vi "ZE_Recorder_CreateTask.vi"(8 "error in":errorcluster, 9 "multi device":bool, 11 "Channel Array In":T1 {"Terminal" items=["Default"=-1, "RSE"=10083, "NRSE"=10078, "Differential"=10106, "Pseudodifferential"=12529]}) -> (0 "error out":errorcluster, 1 "max Range":dbl, 2 "Task Array":refnum<k21>[](array[refnum]), 3 "Channel Array Out":T1 {"Terminal" items=["Default"=-1, "RSE"=10083, "NRSE"=10078, "Differential"=10106, "Pseudodifferential"=12529]})   [LabVIEW 2025, in "ZE_Recorder.lvlib"]
doc: "ZE_Recorder_CreateTask.vi\n----------------------------------------------\nThe VI creates the individual AI or temp tasks and asigns range and teriminal configuration.\nThe channels are assigned to as many tasks as needed.\n\nInputs:\n---------------------\n- error in : Cluster; \n- Channel Array : 1DArrayOfCluster; \n\nOutputs:\n---------------------\n- error out : Cluster; \n- task out : Refnum; \n- Channel Array : 1DArrayOfCluster; \n\n----------------------------------------------\n24.08.2016\nZühlke Engineering AG\nCH-8952 Schlieren\nwww.zuehlke.com"
uses:
  ZE_Recorder.lvlib
  ZE_Recorder_ChannelCluster.ctl
  ChannelCluster.ctl
  ZE_Recorder_Units.ctl
  Temperature.ctl
panel:
  # "Connector Pane"
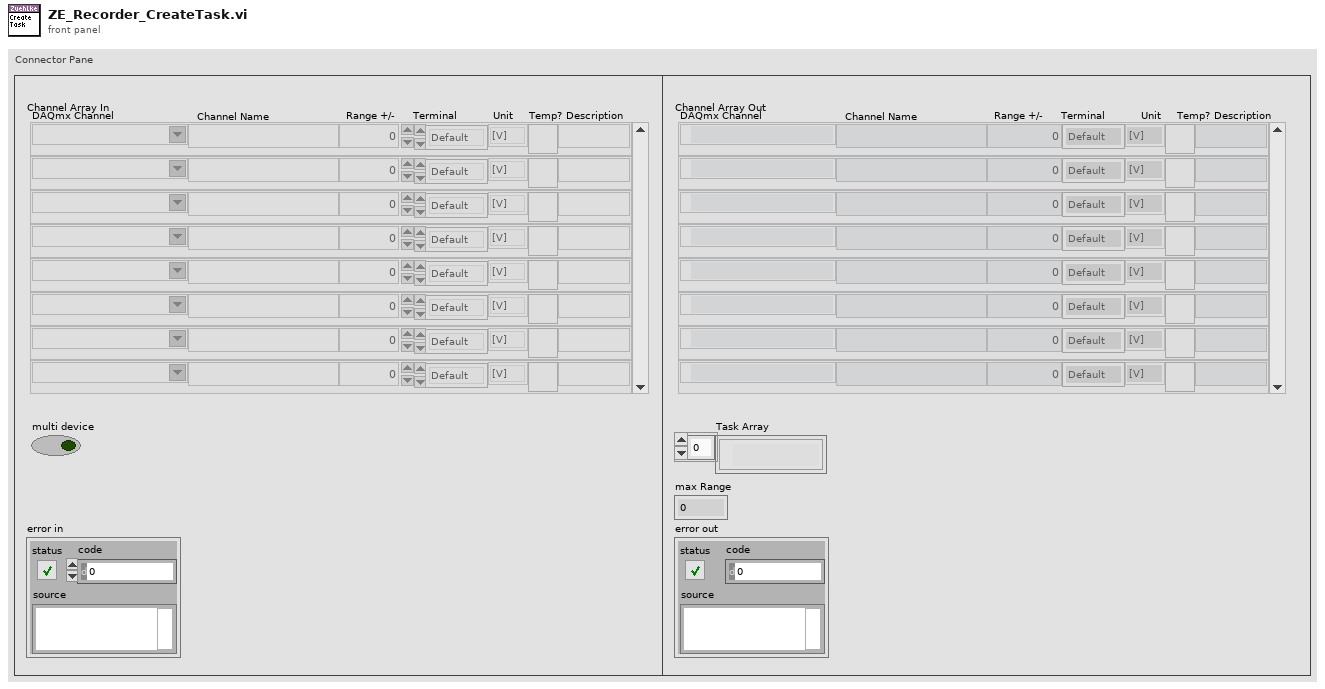
[diagram p1: front panel]
types:
  T1 = typedef "ZE_Recorder.lvlib/ZE_Recorder_ChannelCluster.ctl" = T2[]
  T2 = typedef "ZE_Recorder.lvlib/ChannelCluster.ctl" = cluster{"physical channel":tag, "channel name":string, "Range":dbl, "Terminal":i32, "Unit":T3, "isTemp":T4, "Description":string}
  T3 = typedef "ZE_Recorder.lvlib/ZE_Recorder_Units.ctl" = enum16{"[V]", "[A]", "[F]", "[H]", "[°C]", "[ml/s]", "[m/s]", "[bar]", "[%]", "[N]", "[?]"}
  T4 = typedef "ZE_Recorder.lvlib/Temperature.ctl" = bool
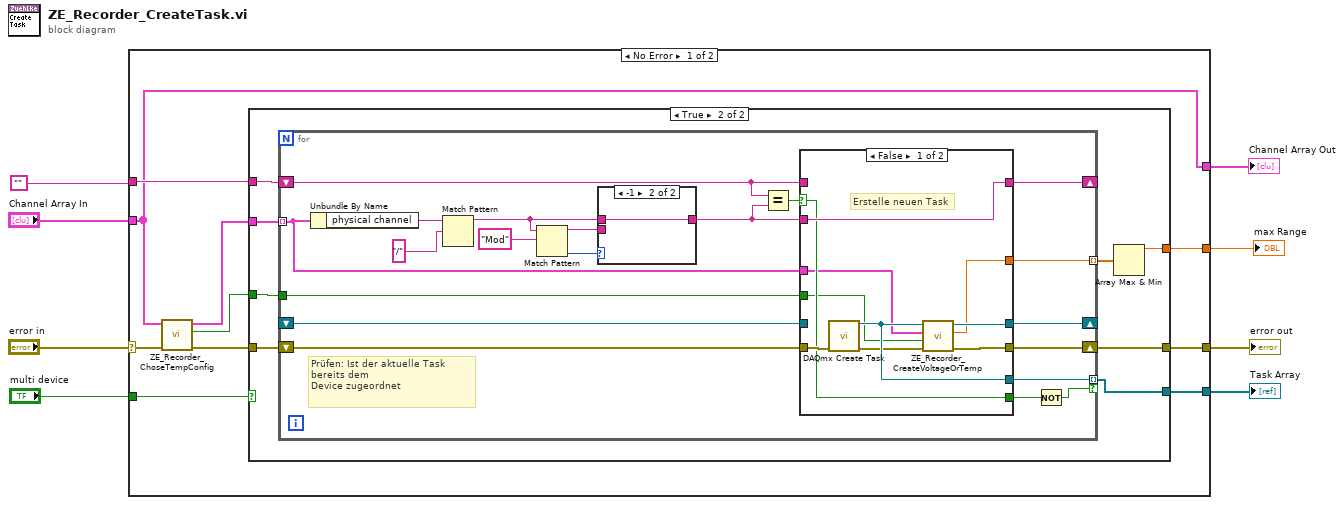
[diagram p0: block diagram]
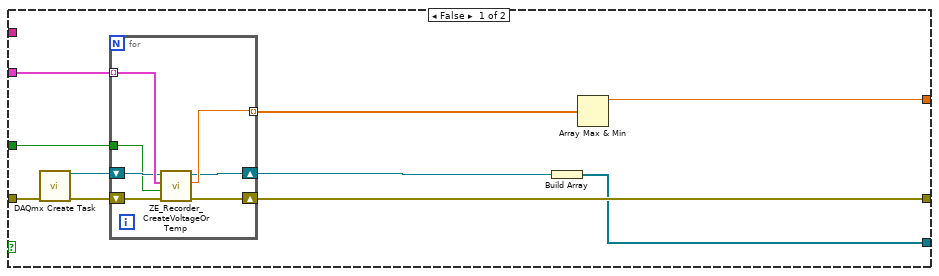
[diagram p2: hidden frame]
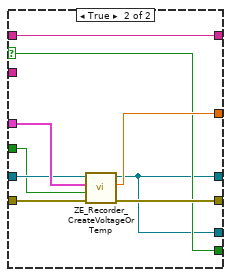
[diagram p4: hidden frame]
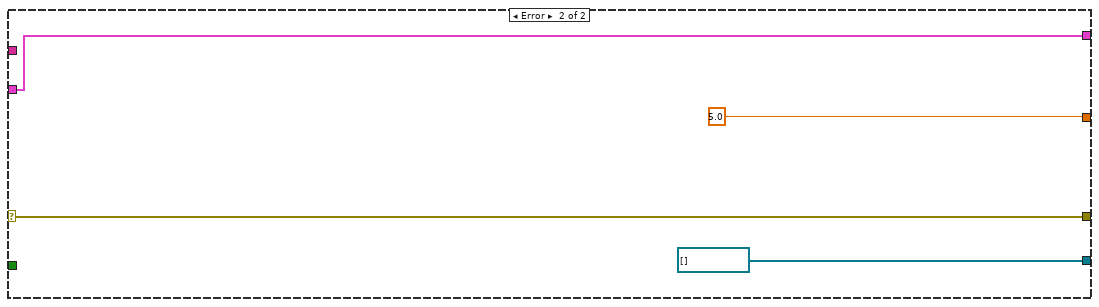
[diagram p5: hidden frame]
diagram:
  n1 = case shown="No Error" "error in" {
    selector: "error in" -> [w11 w87]
    tunnel: "Channel Array In" -> [w13 w88]
    tunnel: [w18 refnum<k21>[] []] -> w5
    tunnel: [w17 w87] -> w6
    tunnel: [w13 w88] -> w4
    tunnel: [w16 5.0] -> w3
    tunnel: "multi device" -> [w15 _]
    tunnel: "" -> [w14 _]
    frame No Error {
      n2 = call "ZE_Recorder_ChoseTempConfig.vi"("error in"=w11, "Channel Array In"=w13) -> ("error out"=w9:errorcluster, "keep config"=w10:bool, "Channel Array out"=w12:T1)  [unwired: 7 in]
      n3 = case shown="True" w15 {
        tunnel: w9 -> [w28 w41]
        tunnel: [w20 w38] -> w18
        tunnel: [w25 w37] -> w17
        tunnel: w12 -> [w24 w43]
        tunnel: [w22 w39] -> w16
        tunnel: w14 -> [_ w42]
        tunnel: w10 -> [w19 w36]
        frame False {
          n4 = call <vilib>:"DAQmx Create Task.vi"("error in"=w28) -> ("task out"=w27:refnum<k21>, "error out"=w26:errorcluster)  [unwired: 13 in]
          n5 = for {
            shift-right: [w30] -> w25
            shift-left: w26 -> [w33]
            shift-right: [w31] -> w21
            shift-left: w27 -> [w34]
            tunnel: w24 -> [w35] mode=indexing
            tunnel: [w32] -> w23 mode=indexing
            tunnel: w19 -> [w29]
            n6 = call "ZE_Recorder_CreateVoltageOrTemp.vi"("Error In"=w33, "keep config?"=w29, "Array Cluster In"=w35, "Task In"=w34) -> ("error out"=w30:errorcluster, "Range (+/-)"=w32:dbl, "Refnum out"=w31:refnum<k21>)  [unwired: 5 in]
          }
          n7 = Build Array(w21) -> (w20:refnum<k21>[])
          n8 = Array Max & Min(array=w23) -> (max value=w22:dbl)  [unwired: 3 out]
        }
        frame True {
          n9 = for {
            tunnel: w43 -> [w58] mode=indexing
            shift-right: [w60] -> _
            shift-left: w42 -> [w53]
            shift-right: [w59] -> _
            shift-left: _ -> [w57]
            shift-right: [w55] -> w37
            shift-left: w41 -> [w56]
            tunnel: [w54] -> w40 mode=indexing
            tunnel: [w52] -> w38 mode=indexing if=w50
            tunnel: w36 -> [w44]
            # "Prüfen: Ist der aktuelle Task bereits dem\nDevice zugeordnet"
            n10 = Unbundle By Name(w58) -> ("physical channel"=w62:tag)
            n11 = Match Pattern(string=w62, regular expression="/") -> (before substring=w46:string)  [unwired: 1 in, 3 out]
            n12 = Match Pattern(string=w46, regular expression="Mod") -> (before substring=w47:string, offset past match=w48:i32)  [unwired: 1 in, 2 out]
            n13 = case shown="-1" w48 {
              tunnel: w47 -> [w64 _]
              tunnel: w46 -> [_ w65]
              tunnel: [w64 w65] -> w45
              frame Default {
              }
              frame -1 {
              }
            }
            n14 = Equal?(x=w53, y=w45) -> (x = y?=w61:bool)
            n15 = case shown="False" w61 {
              selector: w61 -> [w73 w78]
              tunnel: w45 -> [w75 _]
              tunnel: [w75 w79] -> w60
              tunnel: [w69 w77] -> w59
              tunnel: w58 -> [w71 w84]
              tunnel: w57 -> [_ w83]
              tunnel: w56 -> [w74 w82]
              tunnel: [w67 w81] -> w55
              tunnel: [w68 w80] -> w54
              tunnel: w53 -> [_ w79]
              tunnel: [w72 w77] -> w52
              tunnel: [w73 w78] -> w51
              tunnel: w44 -> [w66 w76]
              frame False {
                # "Erstelle neuen Task"
                n16 = call <vilib>:"DAQmx Create Task.vi"("error in"=w74) -> ("task out"=w72:refnum<k21>, "error out"=w70:errorcluster)  [unwired: 13 in]
                n17 = call "ZE_Recorder_CreateVoltageOrTemp.vi"("Error In"=w70, "keep config?"=w66, "Array Cluster In"=w71, "Task In"=w72) -> ("error out"=w67:errorcluster, "Range (+/-)"=w68:dbl, "Refnum out"=w69:refnum<k21>)  [unwired: 5 in]
              }
              frame True {
                n18 = call "ZE_Recorder_CreateVoltageOrTemp.vi"("Error In"=w82, "keep config?"=w76, "Array Cluster In"=w84, "Task In"=w83) -> ("error out"=w81:errorcluster, "Range (+/-)"=w80:dbl, "Refnum out"=w77:refnum<k21>)  [unwired: 5 in]
              }
            }
            n19 = Not(x=w51) -> (.not. x?=w50:bool)
          }
          n20 = Array Max & Min(array=w40) -> (max value=w39:dbl)  [unwired: 3 out]
        }
      }
    }
    frame Error {
    }
  }
  "error out" <- w6
  "Channel Array Out" <- w4
  "max Range" <- w3
  "Task Array" <- w5
